vi "Final_Cell_intra_dcir.vi"(10 "Array in":dbl[](array[numeric]), 11 "L2T":T1) -> (0 "DeltaTcell":bool, 1 "DeltaVcell":bool, 2 "Vcell":bool[](array[boolean]), 3 "Tcell":bool[](array[boolean]), 4 "Dcir":bool)   [LabVIEW 2020]
uses:
  Ctrl/L2T.ctl
panel:
  # "Pre DCIR_____________________________________"
  # "intra DCIR_____________________________________"
  # "Post DCIR_____________________________________"
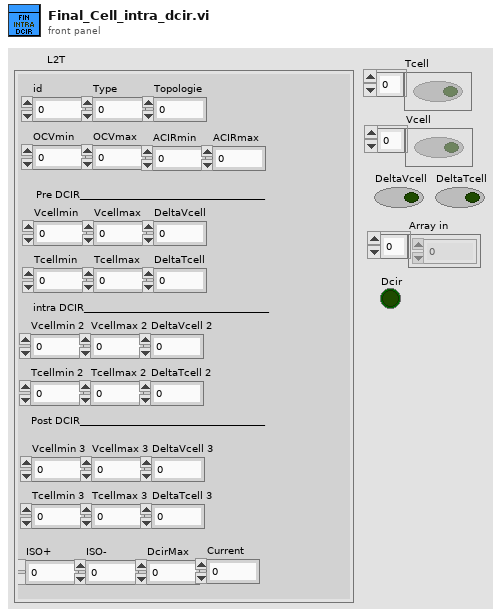
[diagram p1: front panel]
types:
  T1 = typedef "L2T.ctl" = cluster{"id":dbl, "Type":dbl, "OCVmin":dbl, "OCVmax":dbl, "ACIRmin":dbl, "ACIRmax":dbl, "Vcellmin":dbl, "Vcellmax":dbl, "DeltaVcell":dbl, "Tcellmin":dbl, "Tcellmax":dbl, "DeltaTcell":dbl, "ISO+":dbl, "ISO-":dbl, "DcirMax":dbl, "Current":dbl, "Topologie":dbl, "Vcellmin 2":dbl, "Vcellmax 2":dbl, "DeltaVcell 2":dbl, "Tcellmin 2":dbl, "Tcellmax 2":dbl, "DeltaTcell 2":dbl, "Vcellmin 3":dbl, "Vcellmax 3":dbl, "DeltaVcell 3":dbl, "Tcellmin 3":dbl, "Tcellmax 3":dbl, "DeltaTcell 3":dbl}
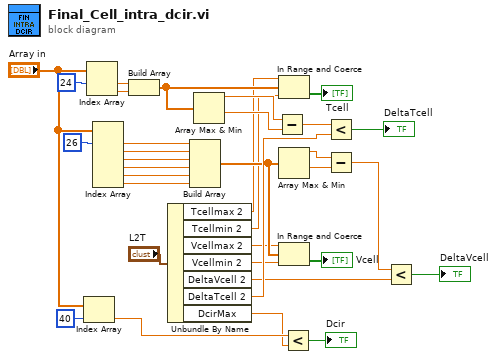
[diagram p0: block diagram]
diagram:
  n1 = Index Array(array="Array in", index=40) -> (element=w3:dbl)
  n2 = Index Array(array="Array in", index #1=24 ("index")) -> (element #1=w25:dbl, element #2=w26:dbl)  [unwired: 1 in]
  n3 = Index Array(array="Array in", index #1=26 ("index")) -> (element #1=w28:dbl, element #2=w29:dbl, element #3=w30:dbl, element #4=w31:dbl, element #5=w32:dbl, element #6=w33:dbl)  [unwired: 5 in]
  n4 = Build Array(w25, w26) -> (w18:dbl[])
  n5 = Unbundle By Name("L2T") -> ("Tcellmax 2"=w6:dbl, "Tcellmin 2"=w7:dbl, "Vcellmax 2"=w8:dbl, "Vcellmin 2"=w9:dbl, "DeltaVcell 2"=w14:dbl, "DeltaTcell 2"=w19:dbl, "DcirMax"=w2:dbl)
  n6 = Build Array(w28, w29, w30, w31, w32, w33) -> (w10:dbl[])
  n7 = Array Max & Min(array=w18) -> (max value=w15:dbl, min value=w16:dbl)  [unwired: 2 out]
  n8 = Subtract(x=w15, y=w16) -> (x-y=w17:dbl)
  n9 = In Range and Coerce ("Dans la gamme")(upper limit=w6, x=w18, lower limit=w7) -> (In Range?=→"Tcell":bool[])  [unwired: 1 out]
  n10 = Array Max & Min(array=w10) -> (max value=w11:dbl, min value=w12:dbl)  [unwired: 2 out]
  n11 = In Range and Coerce ("Dans la gamme")(upper limit=w8, x=w10, lower limit=w9) -> (In Range?=→"Vcell":bool[])  [unwired: 1 out]
  n12 = Less?(x=w3, y=w2) -> (x < y?=→"Dcir":bool)
  n13 = Less?(x=w17, y=w19) -> (x < y?=→"DeltaTcell":bool)
  n14 = Subtract(x=w11, y=w12) -> (x-y=w13:dbl)
  n15 = Less?(x=w13, y=w14) -> (x < y?=→"DeltaVcell":bool)
